vi "create_directory_structure.vi"(1 "Z-stack":bool, 2 "time of last scan":string, 3 "File identifier":string) -> (0 "File path":path)   [LabVIEW 2020]
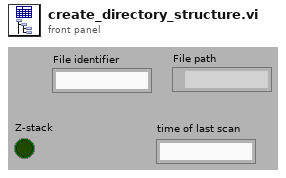
[diagram p1: front panel]
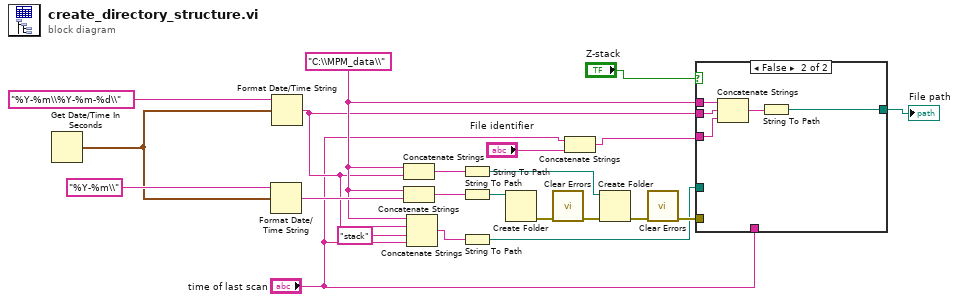
[diagram p0: block diagram]
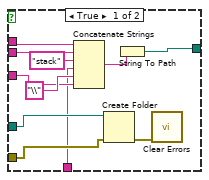
[diagram p2: hidden frame]
diagram:
  w8 = "C:\\MPM_data\\" ("string")
  n1 = Get Date/Time In Seconds() -> (seconds since 1Jan1904=w12:timestamp)
  n2 = Format Date/Time String(time format string (%c)="%Y-%m\\", seconds (now)=w12) -> (date/time string=w20:string)  [unwired: 1 in]
  n3 = Format Date/Time String(time format string (%c)="%Y-%m\\%Y-%m-%d\\", seconds (now)=w12) -> (date/time string=w7:string)  [unwired: 1 in]
  n4 = Concatenate Strings(w8, w7) -> (w21:string)
  n5 = Concatenate Strings(w8, w20) -> (w19:string)
  n6 = Concatenate Strings(w8, w7, "stack" ("string"), "time of last scan") -> (w6:string)
  n7 = String To Path(string=w21) -> (path=w13:path)
  n8 = String To Path(string=w19) -> (path=w14:path)
  n9 = String To Path(string=w6) -> (path=w5:path)
  n10 = Create Folder(path (use dialog)=w14) -> (error out=w17:errorcluster)  [unwired: 2 in, 2 out]
  n11 = call <vilib>:"Clear Errors.vi"("error in (no error)"=w17) -> ("error out"=w15:errorcluster)  [unwired: 5 in, 1 out]
  n12 = Concatenate Strings("time of last scan", "File identifier") -> (w4:string)
  n13 = Create Folder(path (use dialog)=w13, error in=w15) -> (error out=w16:errorcluster)  [unwired: 1 in, 2 out]
  n14 = call <vilib>:"Clear Errors.vi"("error in (no error)"=w16) -> ("error out"=w9:errorcluster)  [unwired: 5 in, 1 out]
  n15 = case shown="False" "Z-stack" {
    tunnel: w7 -> [w33 w38]
    tunnel: w8 -> [w32 w37]
    tunnel: w4 -> [w28 w36]
    tunnel: [w30 w34] -> w11
    tunnel: w9 -> [w26 _]
    tunnel: w5 -> [w25 _]
    tunnel: "time of last scan" -> [w24 _]
    frame True {
      n16 = Concatenate Strings(w32, w33, "stack" ("string"), w24, "\\" ("string"), w28) -> (w31:string)
      n17 = Create Folder(path (use dialog)=w25, error in=w26) -> (error out=w27:errorcluster)  [unwired: 1 in, 2 out]
      n18 = String To Path(string=w31) -> (path=w30:path)
      n19 = call <vilib>:"Clear Errors.vi"("error in (no error)"=w27) -> ()  [unwired: 5 in, 2 out]
    }
    frame False {
      n20 = Concatenate Strings(w37, w38, w36) -> (w35:string)
      n21 = String To Path(string=w35) -> (path=w34:path)
    }
  }
  "File path" <- w11
